vi "Clear Tree.vi"(8 "error in (no error)":errorcluster, 11 "TreeControl in":refnum<vi>) -> (0 "error out":errorcluster)   [LabVIEW 2020, in "DSF Core.lvlib"]
uses:
  DSF Core.lvlib
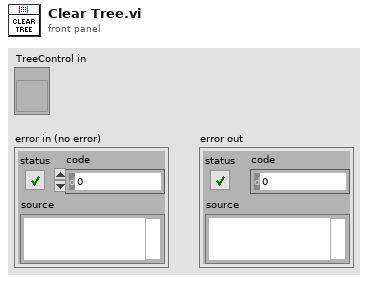
[diagram p1: front panel]
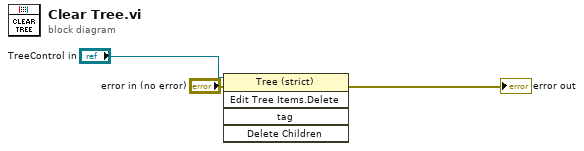
[diagram p0: block diagram]
diagram:
  n1 = invoke class="Tree (strict)" method="Edit Tree Items.Delete"(reference="TreeControl in", error in="error in (no error)") -> (error out=→"error out":errorcluster)  [unwired: 3 in, 4 out]
